vi "Performance Test.vi"() -> ()   [LabVIEW 2021]
uses:
  CIFChannels/Typedef/Direction.ctl
  CIF_NIChn_Fifo_Power.lvclass
  D:/dev/Packages/Channel_Manager/src/CIFChannels/CIFChannels.lvclass
  D:/dev/Packages/Channel_Manager/src/CIF_NIChn/NIChn/CIF_NIChn.lvclass
  ChannelCommon/typedef/FIFO Config.ctl
  <vilib>/Platform/TimedLoop/XDataNode/timing_clust.ctl
  <vilib>/Platform/TimedLoop/XDataNode/nitl_modes.ctl
  <vilib>/Platform/TimedLoop/XDataNode/wakeup.ctl
  ChannelCommon/typedef/Datatype Waveform.ctl
  ChannelCommon/typedef/TimeStamps.ctl
  CIF_NIChn_Fifo_Power.lvclass/CIF_NIChn_Fifo_Power.ctl
  CIFChannels/CIFChannels.lvclass/CIFChannels.ctl
  NIChn/CIF_NIChn.lvclass/CIF_NIChn.ctl
  <vilib>/CIF Foundation/CIF Utilities/DataTypes/Flatten U64.vi
  SubVIs/Add Error.vi
  <vilib>/CIFChannels/Top Level/Write Variable Length U8 Array.vi
  NIChn/Accessors/Read CIF Channel.vi
  NIChn/Accessors/Write CIF Channel.vi
  SubVIs/Flatten.vi
  CIFChannels/Accessors/Read FIFO Payload Length.vi
  NIChn/SubVIs/Check Disconnect.vi
  <vilib>/CIFChannels/Top Level/Read Variable Length U8 Array.vi
  SubVIs/Unflatten.vi
  CIFChannels/Accessors/Read Channel State.vi
  CIFChannels/Accessors/Read Direction.vi
  <vilib>/CIF Foundation/CIF Utilities/Errors/Append Error Location.vi
  <vilib>/CIFChannels/SubVIs/Get dll Path.vi
  ChannelCommon/CIFFIFO/Flatten/Waveform Flatten.vi
  CIFChannels/Accessors/Write Channel State.vi
  CIFChannels/Accessors/Read Tag Disconnect Behavior.vi
  <vilib>/CIFChannels/Top Level/Read Variable Length U8 Array.vi/81056090-23cf-424a-a716-29db01c8ef1b.vi
  <vilib>/CIFChannels/Top Level/Read Variable Length U8 Array.vi/93d598b0-524b-4f76-9570-a74a86ef2c6f.vi
  <vilib>/CIF Foundation/CIF Utilities/DataTypes/Unflatten U64.vi
  ChannelCommon/CIFFIFO/Flatten/Waveform Unflatten.vi
  CIFChannels/Accessors/Write FIFO Header.vi
  CIFChannels/Accessors/Write FIFO Timeout.vi
  <vilib>/CIF Foundation/CIF Utilities/DataTypes/Flatten I64.vi
  ChannelCommon/CIFFIFO/Flatten/Waveform Flatten.vi/be24e584-1bb9-4ddb-b1ad-5fa4498d0a1e.vi
  CIFChannels/Utilities/Create Flattened FIFO Header.vi
  <vilib>/CIFChannels/Top Level/Read Variable Length U8 Array.vi/81056090-23cf-424a-a716-29db01c8ef1b.vi/4bc1c15b-36ab-481f-b8dd-c64075ce723a.vi
  <vilib>/CIFChannels/Top Level/Read Variable Length U8 Array.vi/81056090-23cf-424a-a716-29db01c8ef1b.vi/d83cb72b-7713-41fc-a3d1-682de79cf574.vi
  <vilib>/CIFChannels/Top Level/Read Variable Length U8 Array.vi/93d598b0-524b-4f76-9570-a74a86ef2c6f.vi/4bc1c15b-36ab-481f-b8dd-c64075ce723a.vi
  <vilib>/CIFChannels/Top Level/Read Variable Length U8 Array.vi/93d598b0-524b-4f76-9570-a74a86ef2c6f.vi/d83cb72b-7713-41fc-a3d1-682de79cf574.vi
  ChannelCommon/Utilities/Unflatten Header.vi
  <vilib>/CIF Foundation/CIF Utilities/DataTypes/Unflatten I64.vi
  ChannelCommon/CIFFIFO/Flatten/Waveform Flatten.vi/be24e584-1bb9-4ddb-b1ad-5fa4498d0a1e.vi/c28b0ead-42ad-4072-80a2-aca7f2bd7ce3.vi
  ChannelCommon/Utilities/Flatten Header.vi
  CIFChannels/Utilities/Update FIFO Header.vi
  ChannelCommon/Utilities/Add Error.vi
  <vilib>/CIF Foundation/CIF Utilities/Time/System Time/Get System Time.vi
  <vilib>/CIF Foundation/CIF Utilities/Time/System Time/LabVIEW Time to TAI Time.vi
  NIChn/CIF_NIChn.lvclass
  <vilib>/Platform/TimedLoop/XDataNode/XDataNode.xnode
  <vilib>/Platform/TimedLoop/XDataNode/XDNodeRunTimeDep.lvlib
  CIFChannels/CIFChannels.lvclass
  ChannelCommon/ChannelCommon.lvlib
panel:
  out "avg big channel":dbl
  out "max big channel":dbl
  out "timed out? 4":bool
  out "avg TO":dbl
  out "max TO":dbl
  out "timed out? 3":bool
  out "avg Direct":dbl
  out "max Direct":dbl
  out "timed out? 2":bool
  out "timed out?":bool
  out "avg channel":dbl
  out "max channel":dbl
  out "pass":bool
  out "error out":errorcluster
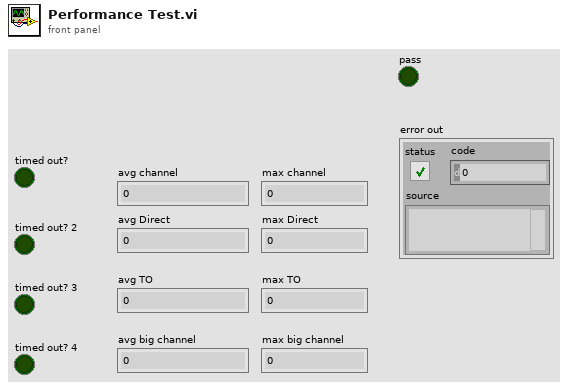
[diagram p1: front panel]
types:
  T1 = typedef "ChannelCommon.lvlib/FIFO Config.ctl" = cluster{"Max Bytes/Msg":u64, "Max Msg/FIFO":u64, "Flags":u64}
  T2 = typedef "CIFChannels.lvclass/Direction.ctl" = enum16{"Publisher", "Subscriber"}
  T3 = typedef "ChannelCommon.lvlib/TimeStamps.ctl" = cluster{"ClockID":u8, "T0":i64, "T_Out":i64}
  T4 = typedef "ChannelCommon.lvlib/Datatype Waveform.ctl" = cluster{"measurement":dbl[], "dT":dbl, "Timestamp":i64, "Read Lock":bool}
  T5 = typedef "XDNodeRunTimeDep.lvlib/timing_clust.ctl" = cluster{"Expected End [f-1]":u64, "Actual End [f-1]":u64, "Finished Late? [f-1]":bool, "Expected End [i-1]":u64, "Actual End [i-1]":u64, "Finished Late? [i-1]":bool, "Expected Start [i]":u64, "Actual Start [i]":u64, "Expected Start [f]":u64, "Actual Start [f]":u64, "Source Name":string, "Structure Name":string, "Period":i64, "Deadline":i64, "Offset":i64, "Start":i64, "Priority":i32, "Timeout":i32, "Mode":T6, "Wakeup Reason":T7, "Error":errorcluster, "Source Type":string, "Secondary Source Type":string, "Global End Time":u64, "Global Start Time":u64, "Frame Duration":u64, "Iteration Duration":u64, "Assigned CPU":i32, "I/O Scan Engine Mode":u32}
  T6 = typedef "XDNodeRunTimeDep.lvlib/nitl_modes.ctl" = enum32{"No Change", "Process missed periods, maintain original phase", "Discard missed periods, maintain original phase", "Process missed periods, ignore original phase", "Discard missed periods, ignore original phase"}
  T7 = typedef "XDNodeRunTimeDep.lvlib/wakeup.ctl" = enum32{"Normal", "Aborted", "Asynchronous wakeup", "Timing source error", "Timed loop error", "Timeout"}
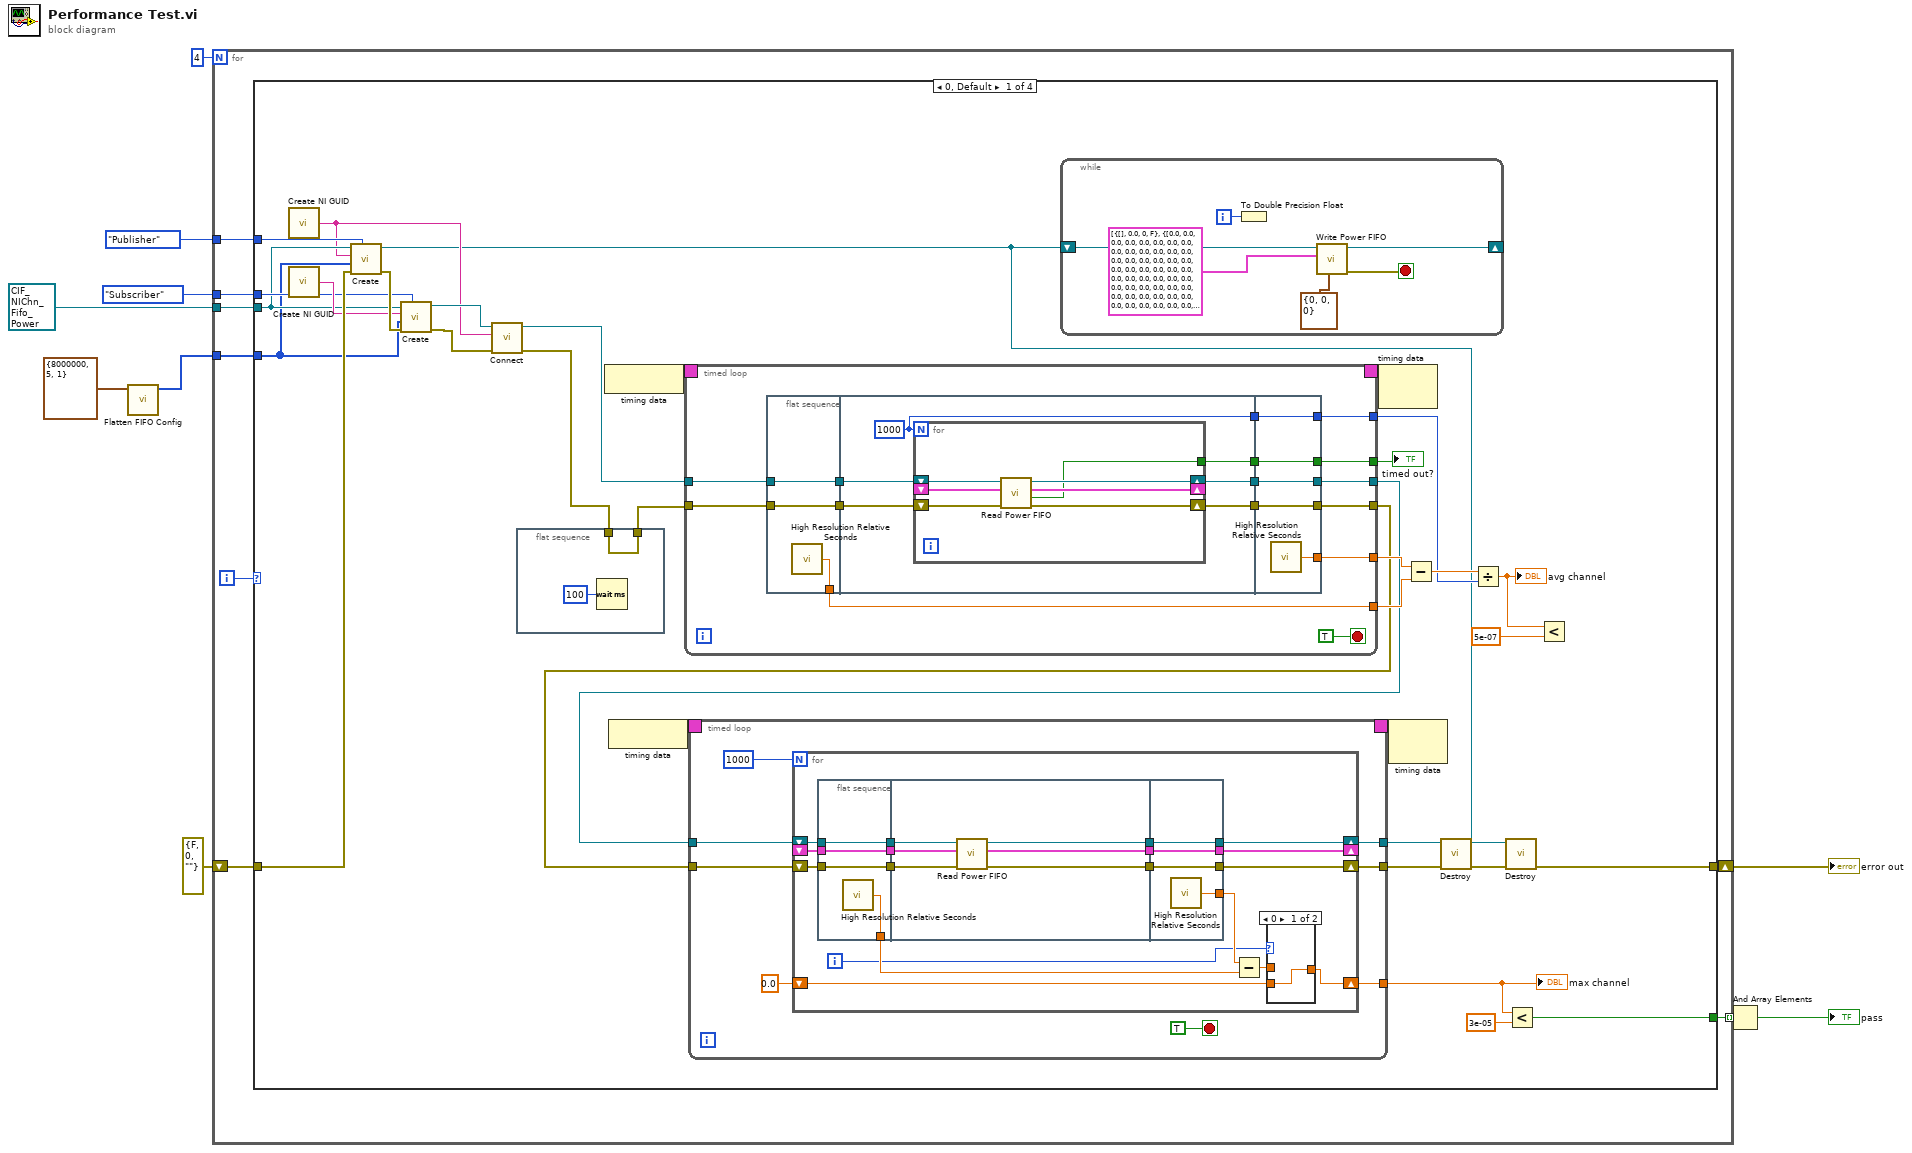
[diagram p0: block diagram]
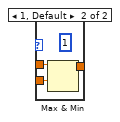
[diagram p2: hidden frame]
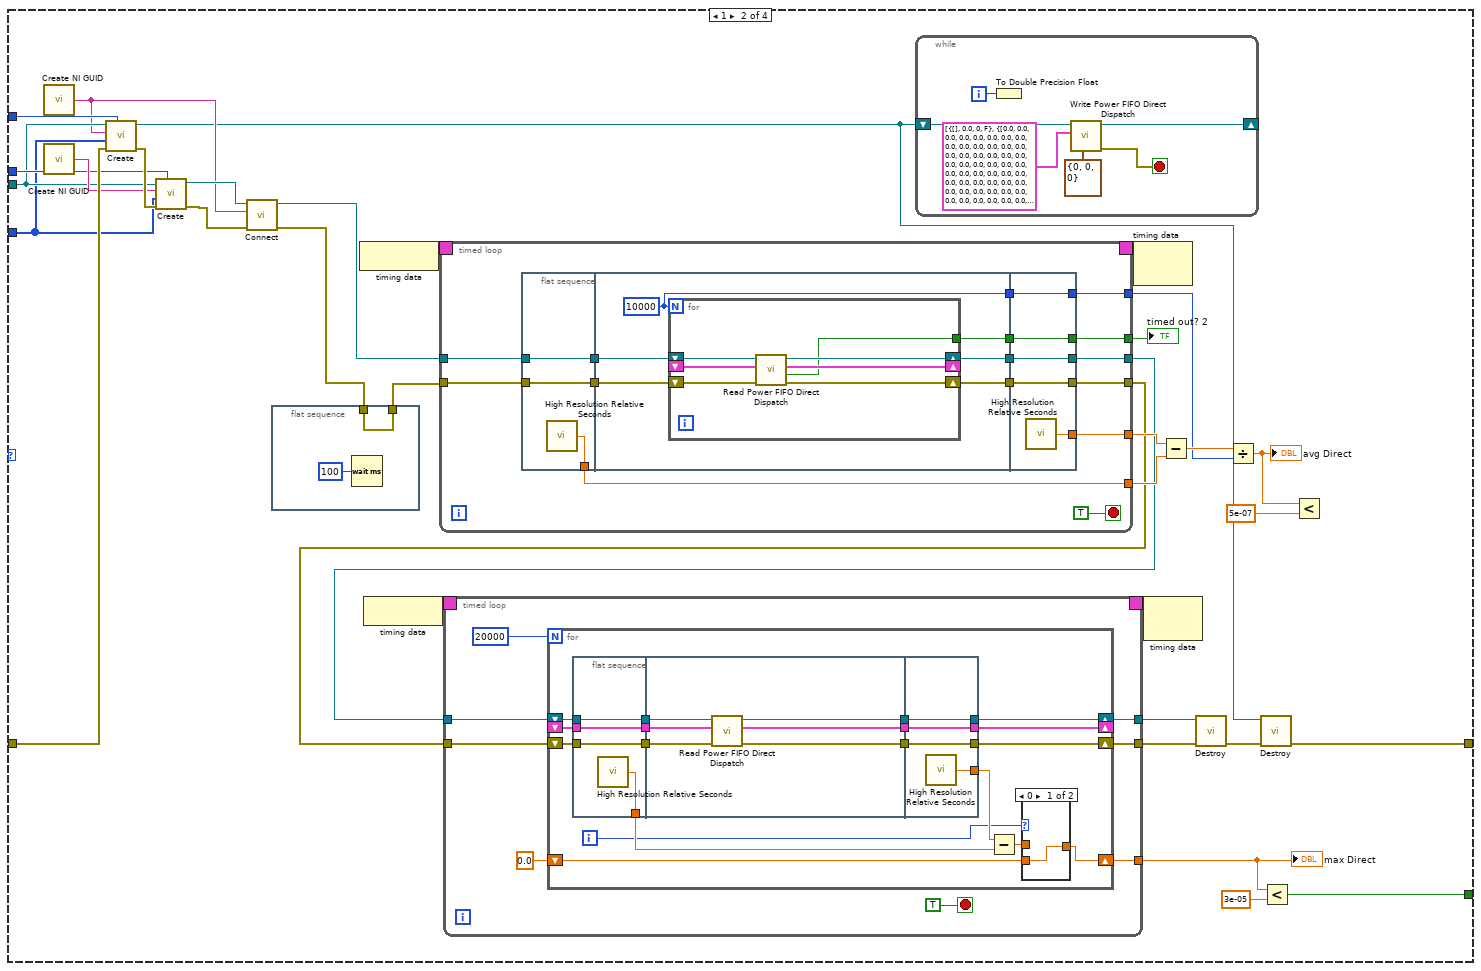
[diagram p3: hidden frame]
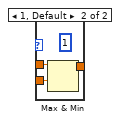
[diagram p4: hidden frame]
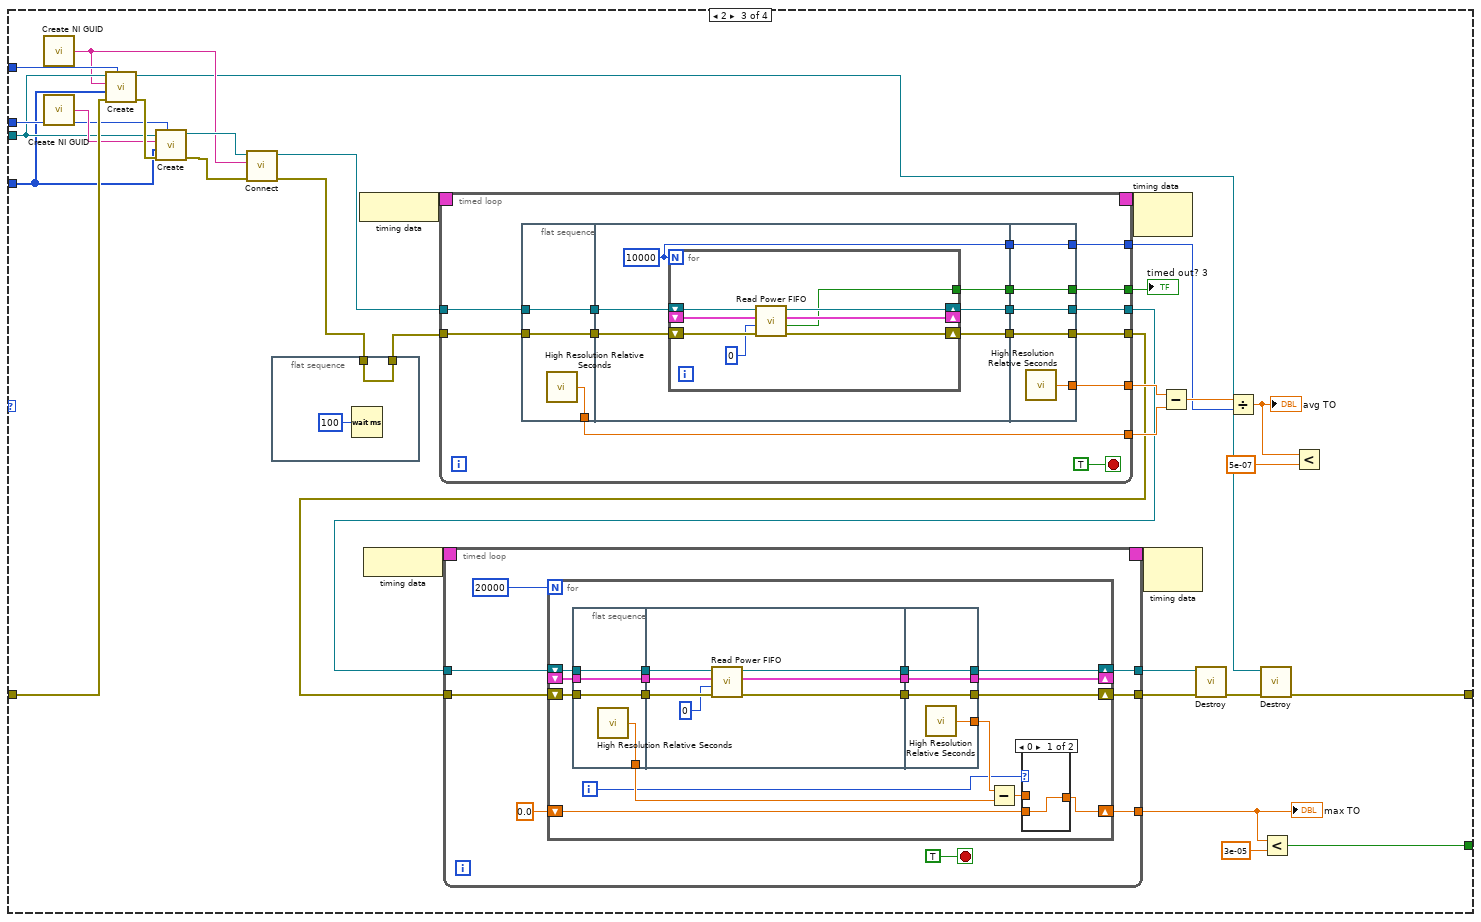
[diagram p5: hidden frame]
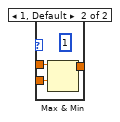
[diagram p6: hidden frame]
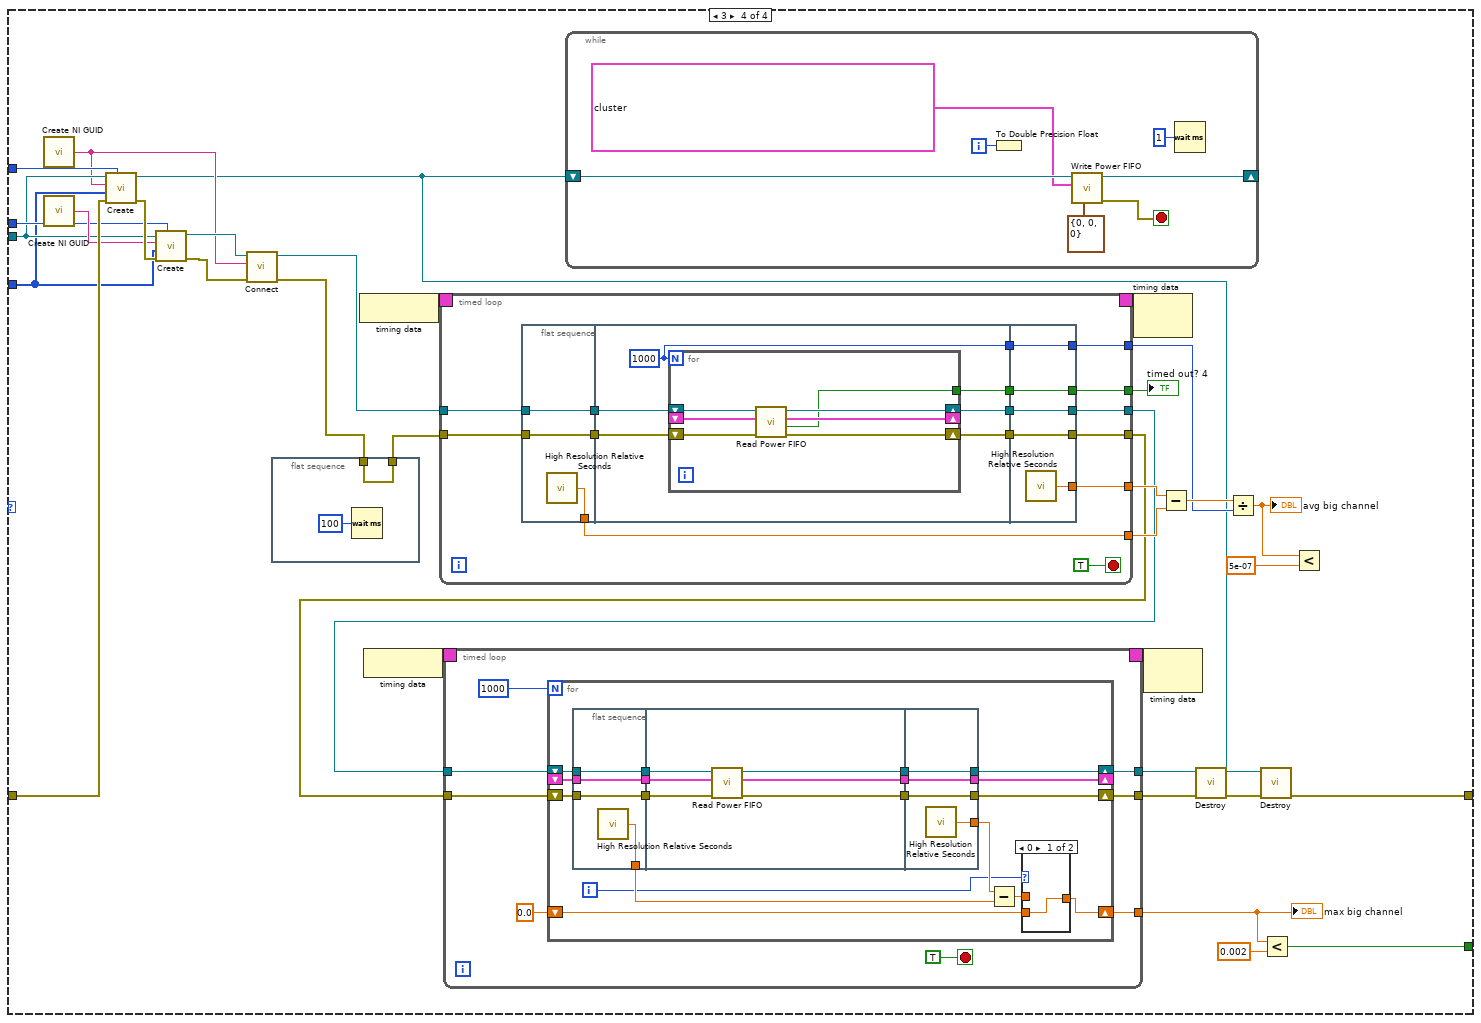
[diagram p7: hidden frame]
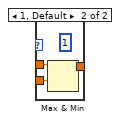
[diagram p8: hidden frame]
diagram:
  n1 = call "Flatten FIFO Config.vi"("FIFO Config in"=T1 {"Max Bytes/Msg"=8000000, "Max Msg/FIFO"=5, "Flags"=1}) -> ("Flattened FIFO Config"=w1:u8[])  [unwired: 10 in]
  n2 = for {
    N: 4 -> [_]
    tunnel: [w18] -> w8 mode=indexing
    shift-right: [w17] -> w10
    shift-left: errorcluster {"status"=FALSE, "code"=0, "source"=""} ("error out") -> [w15]
    tunnel: Direction."Publisher" ("Direction") -> [w14]
    tunnel: Direction."Subscriber" ("Direction") -> [w13]
    tunnel: refnum<class "CIF_NIChn_Fifo_Power.lvclass"> refnum ("CIF_NIChn_Fifo_Power.lvclass") -> [w12]
    tunnel: w1 -> [w11]
    i -> [w16]
    n3 = case shown="0, Default" w16 {
      tunnel: [w38 w168 w298 w424] -> w18
      tunnel: [w22 w152 w282 w408] -> w17
      tunnel: w15 -> [w36 w166 w296 w422]
      tunnel: w14 -> [w34 w164 w294 w420]
      tunnel: w13 -> [w33 w163 w293 w419]
      tunnel: w12 -> [w32 w162 w292 w418]
      tunnel: w11 -> [w28 w158 w288 w414]
      frame 0, Default {
        n4 = call <vilib>:"Create NI GUID.vi"() -> ("NI GUID"=w30:string)
        n5 = call <vilib>:"Create NI GUID.vi"() -> ("NI GUID"=w35:string)
        n6 = call-dynamic "Create.vi"("Direction"=w34, "error in (no error)"=w36, "Custom Config Data"=w28, "Name"=w30, "CIFTag in"=w32) -> ("error out"=w37:errorcluster, "CIFTag out"=w23:refnum<class "CIF_NIChn_Fifo_Power.lvclass">)  [unwired: 5 in]
        n7 = call-dynamic "Create.vi"("Direction"=w33, "error in (no error)"=w37, "Custom Config Data"=w28, "Name"=w35, "CIFTag in"=w32) -> ("error out"=w29:errorcluster, "CIFTag out"=w31:refnum<class "CIF_NIChn_Fifo_Power.lvclass">)  [unwired: 5 in]
        n8 = call-dynamic "Connect.vi"("error in (no error)"=w29, "Connection Name"=w30, "CIFTag in"=w31) -> ("error out"=w21:errorcluster, "CIFTag out"=w27:refnum<class "CIF_NIChn_Fifo_Power.lvclass">)  [unwired: 7 in]
        n9 = flat-sequence {
          tunnel: w21 -> [w54]
          tunnel: [w54] -> w20
          frame #0 {
            n10 = Wait (ms)(milliseconds to wait=u32 100) -> ()  [unwired: 1 out]
          }
        }
        n11 = node-c288() -> (w52:T5)
        n12 = node-c288() -> (w50:T5)
        n13 = timed-loop {
          timing: w52 -> [_]
          timing-out: [_] -> w51
          tunnel: w27 -> [w123]
          tunnel: w20 -> [w122]
          tunnel: [w118] -> w44
          tunnel: [w116] -> w43
          tunnel: [w114] -> w48
          tunnel: [w113] -> w47
          tunnel: [w112] -> w45
          tunnel: [w110] -> w19
          stop <- TRUE stop-if-true
          n14 = flat-sequence {
            tunnel: w122 -> [w125]
            tunnel: w123 -> [w126]
            tunnel: [w126] -> w120
            tunnel: [w125] -> w119
            tunnel: [w124] -> w113
            tunnel: w120 -> [w132]
            tunnel: w119 -> [w131]
            tunnel: [w130] -> w117
            tunnel: [w129] -> w115
            tunnel: [w128] -> w111
            tunnel: [w127] -> w109
            tunnel: [w144] -> w118
            tunnel: w117 -> [w144]
            tunnel: [w143] -> w116
            tunnel: w115 -> [w143]
            tunnel: [w142] -> w114
            tunnel: [w141] -> w112
            tunnel: w111 -> [w141]
            tunnel: [w140] -> w110
            tunnel: w109 -> [w140]
            frame #0 {
              n15 = call <vilib>:"High Resolution Relative Seconds.vi"() -> ("relative seconds"=w124:dbl)
            }
            frame #1 {
              w128 = 1000
              n16 = for {
                N: w128 -> [_]
                shift-right: [w138] -> w130
                shift-left: w132 -> [w139]
                shift-right: [w136] -> w129
                shift-left: w131 -> [w137]
                shift-right: [w135] -> _
                shift-left: _ -> [w133]
                tunnel: [w134] -> w127
                n17 = call-dynamic "Read Power FIFO.vi"("error in (no error)"=w137, "Data in"=w133, "CIFTag in"=w139) -> ("error out"=w136:errorcluster, "timed out?"=w134:bool, "Data out"=w135:T4[], "CIFTag out"=w138:refnum<class "CIF_NIChn_Fifo_Power.lvclass">)  [unwired: 4 in, 1 out]
              }
            }
            frame #2 {
              n18 = call <vilib>:"High Resolution Relative Seconds.vi"() -> ("relative seconds"=w142:dbl)
            }
          }
        }
        "timed out?" <- w19
        n19 = timed-loop {
          timing: w50 -> [_]
          timing-out: [_] -> w49
          tunnel: w44 -> [w68]
          tunnel: w43 -> [w67]
          tunnel: [w65] -> w26
          tunnel: [w64] -> w25
          tunnel: [w61] -> w40
          stop <- TRUE stop-if-true
          n20 = for {
            N: 1000 -> [_]
            shift-right: [w80] -> w65
            shift-left: w68 -> [w82]
            shift-right: [w79] -> w64
            shift-left: w67 -> [w81]
            shift-right: [w73] -> w61
            shift-left: 0.0 -> [w74]
            shift-right: [w72] -> _
            shift-left: _ -> [w78]
            i -> [w70]
            n21 = flat-sequence {
              tunnel: w81 -> [w93]
              tunnel: w82 -> [w94]
              tunnel: [w94] -> w86
              tunnel: [w93] -> w85
              tunnel: [w92] -> w76
              tunnel: w78 -> [w91]
              tunnel: [w91] -> w84
              tunnel: w86 -> [w100]
              tunnel: w85 -> [w98]
              tunnel: [w99] -> w83
              tunnel: w84 -> [w95]
              tunnel: [w96] -> w71
              tunnel: [w97] -> w69
              tunnel: [w104] -> w80
              tunnel: w83 -> [w104]
              tunnel: [w103] -> w79
              tunnel: [w102] -> w77
              tunnel: [w101] -> w72
              tunnel: w71 -> [w101]
              tunnel: w69 -> [w103]
              frame #0 {
                n22 = call <vilib>:"High Resolution Relative Seconds.vi"() -> ("relative seconds"=w92:dbl)
              }
              frame #1 {
                n23 = call-dynamic "Read Power FIFO.vi"("error in (no error)"=w98, "Data in"=w95, "CIFTag in"=w100) -> ("error out"=w97:errorcluster, "Data out"=w96:T4[], "CIFTag out"=w99:refnum<class "CIF_NIChn_Fifo_Power.lvclass">)  [unwired: 4 in, 2 out]
              }
              frame #2 {
                n24 = call <vilib>:"High Resolution Relative Seconds.vi"() -> ("relative seconds"=w102:dbl)
              }
            }
            n25 = Subtract(x=w77, y=w76) -> (x-y=w75:dbl)
            n26 = case shown="0" w70 {
              tunnel: w75 -> [_ w90]
              tunnel: w74 -> [w87 w89]
              tunnel: [w87 w88] -> w73
              frame 0 {
              }
              frame 1, Default {
                (unwired) u32 1 ("milliseconds to wait")
                n27 = Max & Min(x=w90, y=w89) -> (max(x,y)=w88:dbl)  [unwired: 1 out]
              }
            }
          }
        }
        "max channel" <- w40
        n28 = while {
          shift-right: [w55] -> _
          shift-left: w23 -> [w59]
          i -> [w60]
          stop <- w58 stop-if-true
          n29 = To Double Precision Float(number=w60) -> ()  [unwired: 1 out]
          n30 = call-dynamic "Write Power FIFO.vi"("FIFO Timestamps"=T3 {"ClockID"=0, "T0"=0, "T_Out"=0}, "Data In"=T4[] [{"measurement"=[], "dT"=0.0, "Timestamp"=0, "Read Lock"=FALSE}, {"measurement"=[0.0, 0.0, 0.0, 0.0, 0.0, 0.0, 0.0, 0.0, 0.0, 0.0, 0.0, 0.0, 0.0, 0.0, 0.0, 0.0, 0.0, 0.0, 0.0, 0.0, 0.0, 0.0, 0.0, 0.0, 0.0, 0.0, 0.0, 0.0, 0.0, 0.0, 0.0, 0.0, 0.0, 0.0, 0.0, 0.0, 0.0, 0.0, 0.0, 0.0, 0.0, 0.0, 0.0, 0.0, 0.0, 0.0, 0.0, 0.0, 0.0, 0.0, 3.14], "dT"=5.2, "Timestamp"=523, "Read Lock"=FALSE}], "CIFTag in"=w59) -> ("error out"=w58:errorcluster, "CIFTag out"=w55:refnum<class "CIF_NIChn_Fifo_Power.lvclass">)  [unwired: 5 in, 2 out]
        }
        n31 = node-c288(w51) -> ()  [unwired: 1 out]
        n32 = node-c288(w49) -> ()  [unwired: 1 out]
        n33 = Subtract(x=w48, y=w47) -> (x-y=w46:dbl)
        n34 = call-dynamic "Destroy.vi"("error in (no error)"=w25, "CIFTag in"=w26) -> ("error out"=w24:errorcluster)  [unwired: 8 in, 1 out]
        n35 = Divide(x=w46, y=w45) -> (x/y=w42:dbl)
        "avg channel" <- w42
        n36 = call-dynamic "Destroy.vi"("error in (no error)"=w24, "CIFTag in"=w23) -> ("error out"=w22:errorcluster)  [unwired: 8 in, 1 out]
        n37 = Less?(x=w40, y=3e-05) -> (x < y?=w38:bool)
        n38 = Less?(x=w42, y=5e-07) -> ()  [unwired: 1 out]
      }
      frame 1 {
        n39 = call <vilib>:"Create NI GUID.vi"() -> ("NI GUID"=w160:string)
        n40 = call <vilib>:"Create NI GUID.vi"() -> ("NI GUID"=w165:string)
        n41 = call-dynamic "Create.vi"("Direction"=w164, "error in (no error)"=w166, "Custom Config Data"=w158, "Name"=w160, "CIFTag in"=w162) -> ("error out"=w167:errorcluster, "CIFTag out"=w153:refnum<class "CIF_NIChn_Fifo_Power.lvclass">)  [unwired: 5 in]
        n42 = call-dynamic "Create.vi"("Direction"=w163, "error in (no error)"=w167, "Custom Config Data"=w158, "Name"=w165, "CIFTag in"=w162) -> ("error out"=w159:errorcluster, "CIFTag out"=w161:refnum<class "CIF_NIChn_Fifo_Power.lvclass">)  [unwired: 5 in]
        n43 = call-dynamic "Connect.vi"("error in (no error)"=w159, "Connection Name"=w160, "CIFTag in"=w161) -> ("error out"=w151:errorcluster, "CIFTag out"=w157:refnum<class "CIF_NIChn_Fifo_Power.lvclass">)  [unwired: 7 in]
        n44 = flat-sequence {
          tunnel: w151 -> [w184]
          tunnel: [w184] -> w150
          frame #0 {
            n45 = Wait (ms)(milliseconds to wait=u32 100) -> ()  [unwired: 1 out]
          }
        }
        n46 = node-c288() -> (w182:T5)
        n47 = node-c288() -> (w180:T5)
        n48 = timed-loop {
          timing: w182 -> [_]
          timing-out: [_] -> w181
          tunnel: w157 -> [w253]
          tunnel: w150 -> [w252]
          tunnel: [w248] -> w174
          tunnel: [w246] -> w173
          tunnel: [w244] -> w178
          tunnel: [w243] -> w177
          tunnel: [w242] -> w175
          tunnel: [w240] -> w149
          stop <- TRUE stop-if-true
          n49 = flat-sequence {
            tunnel: w252 -> [w255]
            tunnel: w253 -> [w256]
            tunnel: [w256] -> w250
            tunnel: [w255] -> w249
            tunnel: [w254] -> w243
            tunnel: w250 -> [w262]
            tunnel: w249 -> [w261]
            tunnel: [w260] -> w247
            tunnel: [w259] -> w245
            tunnel: [w258] -> w241
            tunnel: [w257] -> w239
            tunnel: [w274] -> w248
            tunnel: w247 -> [w274]
            tunnel: [w273] -> w246
            tunnel: w245 -> [w273]
            tunnel: [w272] -> w244
            tunnel: [w271] -> w242
            tunnel: w241 -> [w271]
            tunnel: [w270] -> w240
            tunnel: w239 -> [w270]
            frame #0 {
              n50 = call <vilib>:"High Resolution Relative Seconds.vi"() -> ("relative seconds"=w254:dbl)
            }
            frame #1 {
              w258 = 10000
              n51 = for {
                N: w258 -> [_]
                shift-right: [w268] -> w260
                shift-left: w262 -> [w269]
                shift-right: [w266] -> w259
                shift-left: w261 -> [w267]
                shift-right: [w265] -> _
                shift-left: _ -> [w263]
                tunnel: [w264] -> w257
                n52 = call "Read Power FIFO Direct Dispatch.vi"("error in (no error)"=w267, "Data in"=w263, "CIFTag in"=w269) -> ("error out"=w266:errorcluster, "timed out?"=w264:bool, "Data out"=w265:T4[], "CIFTag out"=w268:refnum<class "CIF_NIChn_Fifo_Power.lvclass">)  [unwired: 4 in, 1 out]
              }
            }
            frame #2 {
              n53 = call <vilib>:"High Resolution Relative Seconds.vi"() -> ("relative seconds"=w272:dbl)
            }
          }
        }
        "timed out? 2" <- w149
        n54 = timed-loop {
          timing: w180 -> [_]
          timing-out: [_] -> w179
          tunnel: w174 -> [w198]
          tunnel: w173 -> [w197]
          tunnel: [w195] -> w156
          tunnel: [w194] -> w155
          tunnel: [w191] -> w170
          stop <- TRUE stop-if-true
          n55 = for {
            N: 20000 -> [_]
            shift-right: [w210] -> w195
            shift-left: w198 -> [w212]
            shift-right: [w209] -> w194
            shift-left: w197 -> [w211]
            shift-right: [w203] -> w191
            shift-left: 0.0 -> [w204]
            shift-right: [w202] -> _
            shift-left: _ -> [w208]
            i -> [w200]
            n56 = flat-sequence {
              tunnel: w211 -> [w223]
              tunnel: w212 -> [w224]
              tunnel: [w224] -> w216
              tunnel: [w223] -> w215
              tunnel: [w222] -> w206
              tunnel: w208 -> [w221]
              tunnel: [w221] -> w214
              tunnel: w216 -> [w230]
              tunnel: w215 -> [w228]
              tunnel: [w229] -> w213
              tunnel: w214 -> [w225]
              tunnel: [w226] -> w201
              tunnel: [w227] -> w199
              tunnel: [w234] -> w210
              tunnel: w213 -> [w234]
              tunnel: [w233] -> w209
              tunnel: [w232] -> w207
              tunnel: [w231] -> w202
              tunnel: w201 -> [w231]
              tunnel: w199 -> [w233]
              frame #0 {
                n57 = call <vilib>:"High Resolution Relative Seconds.vi"() -> ("relative seconds"=w222:dbl)
              }
              frame #1 {
                n58 = call "Read Power FIFO Direct Dispatch.vi"("error in (no error)"=w228, "Data in"=w225, "CIFTag in"=w230) -> ("error out"=w227:errorcluster, "Data out"=w226:T4[], "CIFTag out"=w229:refnum<class "CIF_NIChn_Fifo_Power.lvclass">)  [unwired: 4 in, 2 out]
              }
              frame #2 {
                n59 = call <vilib>:"High Resolution Relative Seconds.vi"() -> ("relative seconds"=w232:dbl)
              }
            }
            n60 = Subtract(x=w207, y=w206) -> (x-y=w205:dbl)
            n61 = case shown="0" w200 {
              tunnel: w205 -> [_ w220]
              tunnel: w204 -> [w217 w219]
              tunnel: [w217 w218] -> w203
              frame 0 {
              }
              frame 1, Default {
                (unwired) u32 1 ("milliseconds to wait")
                n62 = Max & Min(x=w220, y=w219) -> (max(x,y)=w218:dbl)  [unwired: 1 out]
              }
            }
          }
        }
        "max Direct" <- w170
        n63 = while {
          shift-right: [w185] -> _
          shift-left: w153 -> [w189]
          i -> [w190]
          stop <- w188 stop-if-true
          n64 = To Double Precision Float(number=w190) -> ()  [unwired: 1 out]
          n65 = call "Write Power FIFO Direct Dispatch.vi"("FIFO Timestamps"=T3 {"ClockID"=0, "T0"=0, "T_Out"=0}, "Data In"=T4[] [{"measurement"=[], "dT"=0.0, "Timestamp"=0, "Read Lock"=FALSE}, {"measurement"=[0.0, 0.0, 0.0, 0.0, 0.0, 0.0, 0.0, 0.0, 0.0, 0.0, 0.0, 0.0, 0.0, 0.0, 0.0, 0.0, 0.0, 0.0, 0.0, 0.0, 0.0, 0.0, 0.0, 0.0, 0.0, 0.0, 0.0, 0.0, 0.0, 0.0, 0.0, 0.0, 0.0, 0.0, 0.0, 0.0, 0.0, 0.0, 0.0, 0.0, 0.0, 0.0, 0.0, 0.0, 0.0, 0.0, 0.0, 0.0, 0.0, 0.0, 3.14], "dT"=5.2, "Timestamp"=523, "Read Lock"=FALSE}], "CIFTag in"=w189) -> ("error out"=w188:errorcluster, "CIFTag out"=w185:refnum<class "CIF_NIChn_Fifo_Power.lvclass">)  [unwired: 5 in, 2 out]
        }
        n66 = node-c288(w181) -> ()  [unwired: 1 out]
        n67 = node-c288(w179) -> ()  [unwired: 1 out]
        n68 = Subtract(x=w178, y=w177) -> (x-y=w176:dbl)
        n69 = call-dynamic "Destroy.vi"("error in (no error)"=w155, "CIFTag in"=w156) -> ("error out"=w154:errorcluster)  [unwired: 8 in, 1 out]
        n70 = Divide(x=w176, y=w175) -> (x/y=w172:dbl)
        "avg Direct" <- w172
        n71 = call-dynamic "Destroy.vi"("error in (no error)"=w154, "CIFTag in"=w153) -> ("error out"=w152:errorcluster)  [unwired: 8 in, 1 out]
        n72 = Less?(x=w170, y=3e-05) -> (x < y?=w168:bool)
        n73 = Less?(x=w172, y=5e-07) -> ()  [unwired: 1 out]
      }
      frame 2 {
        n74 = call <vilib>:"Create NI GUID.vi"() -> ("NI GUID"=w290:string)
        n75 = call <vilib>:"Create NI GUID.vi"() -> ("NI GUID"=w295:string)
        n76 = call-dynamic "Create.vi"("Direction"=w294, "error in (no error)"=w296, "Custom Config Data"=w288, "Name"=w290, "CIFTag in"=w292) -> ("error out"=w297:errorcluster, "CIFTag out"=w283:refnum<class "CIF_NIChn_Fifo_Power.lvclass">)  [unwired: 5 in]
        n77 = call-dynamic "Create.vi"("Direction"=w293, "error in (no error)"=w297, "Custom Config Data"=w288, "Name"=w295, "CIFTag in"=w292) -> ("error out"=w289:errorcluster, "CIFTag out"=w291:refnum<class "CIF_NIChn_Fifo_Power.lvclass">)  [unwired: 5 in]
        n78 = call-dynamic "Connect.vi"("error in (no error)"=w289, "Connection Name"=w290, "CIFTag in"=w291) -> ("error out"=w281:errorcluster, "CIFTag out"=w287:refnum<class "CIF_NIChn_Fifo_Power.lvclass">)  [unwired: 7 in]
        n79 = flat-sequence {
          tunnel: w281 -> [w314]
          tunnel: [w314] -> w280
          frame #0 {
            n80 = Wait (ms)(milliseconds to wait=u32 100) -> ()  [unwired: 1 out]
          }
        }
        n81 = node-c288() -> (w312:T5)
        n82 = node-c288() -> (w310:T5)
        n83 = timed-loop {
          timing: w312 -> [_]
          timing-out: [_] -> w311
          tunnel: w287 -> [w378]
          tunnel: w280 -> [w377]
          tunnel: [w373] -> w304
          tunnel: [w371] -> w303
          tunnel: [w369] -> w308
          tunnel: [w368] -> w307
          tunnel: [w367] -> w305
          tunnel: [w365] -> w279
          stop <- TRUE stop-if-true
          n84 = flat-sequence {
            tunnel: w377 -> [w380]
            tunnel: w378 -> [w381]
            tunnel: [w381] -> w375
            tunnel: [w380] -> w374
            tunnel: [w379] -> w368
            tunnel: w375 -> [w387]
            tunnel: w374 -> [w386]
            tunnel: [w385] -> w372
            tunnel: [w384] -> w370
            tunnel: [w383] -> w366
            tunnel: [w382] -> w364
            tunnel: [w400] -> w373
            tunnel: w372 -> [w400]
            tunnel: [w399] -> w371
            tunnel: w370 -> [w399]
            tunnel: [w398] -> w369
            tunnel: [w397] -> w367
            tunnel: w366 -> [w397]
            tunnel: [w396] -> w365
            tunnel: w364 -> [w396]
            frame #0 {
              n85 = call <vilib>:"High Resolution Relative Seconds.vi"() -> ("relative seconds"=w379:dbl)
            }
            frame #1 {
              w383 = 10000
              n86 = for {
                N: w383 -> [_]
                shift-right: [w394] -> w385
                shift-left: w387 -> [w395]
                shift-right: [w392] -> w384
                shift-left: w386 -> [w393]
                shift-right: [w391] -> _
                shift-left: _ -> [w388]
                tunnel: [w390] -> w382
                n87 = call-dynamic "Read Power FIFO.vi"("error in (no error)"=w393, "Timeout (ms)"=0, "Data in"=w388, "CIFTag in"=w395) -> ("error out"=w392:errorcluster, "timed out?"=w390:bool, "Data out"=w391:T4[], "CIFTag out"=w394:refnum<class "CIF_NIChn_Fifo_Power.lvclass">)  [unwired: 3 in, 1 out]
              }
            }
            frame #2 {
              n88 = call <vilib>:"High Resolution Relative Seconds.vi"() -> ("relative seconds"=w398:dbl)
            }
          }
        }
        "timed out? 3" <- w279
        n89 = timed-loop {
          timing: w310 -> [_]
          timing-out: [_] -> w309
          tunnel: w304 -> [w322]
          tunnel: w303 -> [w321]
          tunnel: [w319] -> w286
          tunnel: [w318] -> w285
          tunnel: [w315] -> w300
          stop <- TRUE stop-if-true
          n90 = for {
            N: 20000 -> [_]
            shift-right: [w334] -> w319
            shift-left: w322 -> [w336]
            shift-right: [w333] -> w318
            shift-left: w321 -> [w335]
            shift-right: [w327] -> w315
            shift-left: 0.0 -> [w328]
            shift-right: [w326] -> _
            shift-left: _ -> [w332]
            i -> [w324]
            n91 = flat-sequence {
              tunnel: w335 -> [w347]
              tunnel: w336 -> [w348]
              tunnel: [w348] -> w340
              tunnel: [w347] -> w339
              tunnel: [w346] -> w330
              tunnel: w332 -> [w345]
              tunnel: [w345] -> w338
              tunnel: w340 -> [w355]
              tunnel: w339 -> [w353]
              tunnel: [w354] -> w337
              tunnel: w338 -> [w349]
              tunnel: [w351] -> w325
              tunnel: [w352] -> w323
              tunnel: [w359] -> w334
              tunnel: w337 -> [w359]
              tunnel: [w358] -> w333
              tunnel: [w357] -> w331
              tunnel: [w356] -> w326
              tunnel: w325 -> [w356]
              tunnel: w323 -> [w358]
              frame #0 {
                n92 = call <vilib>:"High Resolution Relative Seconds.vi"() -> ("relative seconds"=w346:dbl)
              }
              frame #1 {
                n93 = call-dynamic "Read Power FIFO.vi"("error in (no error)"=w353, "Timeout (ms)"=0, "Data in"=w349, "CIFTag in"=w355) -> ("error out"=w352:errorcluster, "Data out"=w351:T4[], "CIFTag out"=w354:refnum<class "CIF_NIChn_Fifo_Power.lvclass">)  [unwired: 3 in, 2 out]
              }
              frame #2 {
                n94 = call <vilib>:"High Resolution Relative Seconds.vi"() -> ("relative seconds"=w357:dbl)
              }
            }
            n95 = Subtract(x=w331, y=w330) -> (x-y=w329:dbl)
            n96 = case shown="0" w324 {
              tunnel: w329 -> [_ w344]
              tunnel: w328 -> [w341 w343]
              tunnel: [w341 w342] -> w327
              frame 0 {
              }
              frame 1, Default {
                (unwired) u32 1 ("milliseconds to wait")
                n97 = Max & Min(x=w344, y=w343) -> (max(x,y)=w342:dbl)  [unwired: 1 out]
              }
            }
          }
        }
        "max TO" <- w300
        n98 = node-c288(w311) -> ()  [unwired: 1 out]
        n99 = node-c288(w309) -> ()  [unwired: 1 out]
        n100 = Subtract(x=w308, y=w307) -> (x-y=w306:dbl)
        n101 = call-dynamic "Destroy.vi"("error in (no error)"=w285, "CIFTag in"=w286) -> ("error out"=w284:errorcluster)  [unwired: 8 in, 1 out]
        n102 = Divide(x=w306, y=w305) -> (x/y=w302:dbl)
        "avg TO" <- w302
        n103 = call-dynamic "Destroy.vi"("error in (no error)"=w284, "CIFTag in"=w283) -> ("error out"=w282:errorcluster)  [unwired: 8 in, 1 out]
        n104 = Less?(x=w300, y=3e-05) -> (x < y?=w298:bool)
        n105 = Less?(x=w302, y=5e-07) -> ()  [unwired: 1 out]
      }
      frame 3 {
        n106 = call <vilib>:"Create NI GUID.vi"() -> ("NI GUID"=w416:string)
        n107 = call <vilib>:"Create NI GUID.vi"() -> ("NI GUID"=w421:string)
        n108 = call-dynamic "Create.vi"("Direction"=w420, "error in (no error)"=w422, "Custom Config Data"=w414, "Name"=w416, "CIFTag in"=w418) -> ("error out"=w423:errorcluster, "CIFTag out"=w409:refnum<class "CIF_NIChn_Fifo_Power.lvclass">)  [unwired: 5 in]
        n109 = call-dynamic "Create.vi"("Direction"=w419, "error in (no error)"=w423, "Custom Config Data"=w414, "Name"=w421, "CIFTag in"=w418) -> ("error out"=w415:errorcluster, "CIFTag out"=w417:refnum<class "CIF_NIChn_Fifo_Power.lvclass">)  [unwired: 5 in]
        n110 = call-dynamic "Connect.vi"("error in (no error)"=w415, "Connection Name"=w416, "CIFTag in"=w417) -> ("error out"=w407:errorcluster, "CIFTag out"=w413:refnum<class "CIF_NIChn_Fifo_Power.lvclass">)  [unwired: 7 in]
        n111 = flat-sequence {
          tunnel: w407 -> [w440]
          tunnel: [w440] -> w406
          frame #0 {
            n112 = Wait (ms)(milliseconds to wait=u32 100) -> ()  [unwired: 1 out]
          }
        }
        n113 = node-c288() -> (w438:T5)
        n114 = node-c288() -> (w436:T5)
        n115 = timed-loop {
          timing: w438 -> [_]
          timing-out: [_] -> w437
          tunnel: w413 -> [w510]
          tunnel: w406 -> [w509]
          tunnel: [w505] -> w430
          tunnel: [w503] -> w429
          tunnel: [w501] -> w434
          tunnel: [w500] -> w433
          tunnel: [w499] -> w431
          tunnel: [w497] -> w405
          stop <- TRUE stop-if-true
          n116 = flat-sequence {
            tunnel: w509 -> [w512]
            tunnel: w510 -> [w513]
            tunnel: [w513] -> w507
            tunnel: [w512] -> w506
            tunnel: [w511] -> w500
            tunnel: w507 -> [w519]
            tunnel: w506 -> [w518]
            tunnel: [w517] -> w504
            tunnel: [w516] -> w502
            tunnel: [w515] -> w498
            tunnel: [w514] -> w496
            tunnel: [w531] -> w505
            tunnel: w504 -> [w531]
            tunnel: [w530] -> w503
            tunnel: w502 -> [w530]
            tunnel: [w529] -> w501
            tunnel: [w528] -> w499
            tunnel: w498 -> [w528]
            tunnel: [w527] -> w497
            tunnel: w496 -> [w527]
            frame #0 {
              n117 = call <vilib>:"High Resolution Relative Seconds.vi"() -> ("relative seconds"=w511:dbl)
            }
            frame #1 {
              w515 = 1000
              n118 = for {
                N: w515 -> [_]
                shift-right: [w525] -> w517
                shift-left: w519 -> [w526]
                shift-right: [w523] -> w516
                shift-left: w518 -> [w524]
                shift-right: [w522] -> _
                shift-left: _ -> [w520]
                tunnel: [w521] -> w514
                n119 = call-dynamic "Read Power FIFO.vi"("error in (no error)"=w524, "Data in"=w520, "CIFTag in"=w526) -> ("error out"=w523:errorcluster, "timed out?"=w521:bool, "Data out"=w522:T4[], "CIFTag out"=w525:refnum<class "CIF_NIChn_Fifo_Power.lvclass">)  [unwired: 4 in, 1 out]
              }
            }
            frame #2 {
              n120 = call <vilib>:"High Resolution Relative Seconds.vi"() -> ("relative seconds"=w529:dbl)
            }
          }
        }
        "timed out? 4" <- w405
        n121 = timed-loop {
          timing: w436 -> [_]
          timing-out: [_] -> w435
          tunnel: w430 -> [w455]
          tunnel: w429 -> [w454]
          tunnel: [w452] -> w412
          tunnel: [w451] -> w411
          tunnel: [w448] -> w426
          stop <- TRUE stop-if-true
          n122 = for {
            N: 1000 -> [_]
            shift-right: [w467] -> w452
            shift-left: w455 -> [w469]
            shift-right: [w466] -> w451
            shift-left: w454 -> [w468]
            shift-right: [w460] -> w448
            shift-left: 0.0 -> [w461]
            shift-right: [w459] -> _
            shift-left: _ -> [w465]
            i -> [w457]
            n123 = flat-sequence {
              tunnel: w468 -> [w480]
              tunnel: w469 -> [w481]
              tunnel: [w481] -> w473
              tunnel: [w480] -> w472
              tunnel: [w479] -> w463
              tunnel: w465 -> [w478]
              tunnel: [w478] -> w471
              tunnel: w473 -> [w487]
              tunnel: w472 -> [w485]
              tunnel: [w486] -> w470
              tunnel: w471 -> [w482]
              tunnel: [w483] -> w458
              tunnel: [w484] -> w456
              tunnel: [w491] -> w467
              tunnel: w470 -> [w491]
              tunnel: [w490] -> w466
              tunnel: [w489] -> w464
              tunnel: [w488] -> w459
              tunnel: w458 -> [w488]
              tunnel: w456 -> [w490]
              frame #0 {
                n124 = call <vilib>:"High Resolution Relative Seconds.vi"() -> ("relative seconds"=w479:dbl)
              }
              frame #1 {
                n125 = call-dynamic "Read Power FIFO.vi"("error in (no error)"=w485, "Data in"=w482, "CIFTag in"=w487) -> ("error out"=w484:errorcluster, "Data out"=w483:T4[], "CIFTag out"=w486:refnum<class "CIF_NIChn_Fifo_Power.lvclass">)  [unwired: 4 in, 2 out]
              }
              frame #2 {
                n126 = call <vilib>:"High Resolution Relative Seconds.vi"() -> ("relative seconds"=w489:dbl)
              }
            }
            n127 = Subtract(x=w464, y=w463) -> (x-y=w462:dbl)
            n128 = case shown="0" w457 {
              tunnel: w462 -> [_ w477]
              tunnel: w461 -> [w474 w476]
              tunnel: [w474 w475] -> w460
              frame 0 {
              }
              frame 1, Default {
                (unwired) u32 1 ("milliseconds to wait")
                n129 = Max & Min(x=w477, y=w476) -> (max(x,y)=w475:dbl)  [unwired: 1 out]
              }
            }
          }
        }
        "max big channel" <- w426
        n130 = while {
          shift-right: [w441] -> _
          shift-left: w409 -> [w446]
          i -> [w447]
          stop <- w445 stop-if-true
          n131 = To Double Precision Float(number=w447) -> ()  [unwired: 1 out]
          n132 = call-dynamic "Write Power FIFO.vi"("FIFO Timestamps"=T3 {"ClockID"=0, "T0"=0, "T_Out"=0}, "Data In"=T4[] [{"measurement"=array[200001 elements], "dT"=0.0, "Timestamp"=0, "Read Lock"=FALSE}, {"measurement"=array[200001 elements], "dT"=5.2, "Timestamp"=523, "Read Lock"=FALSE}], "CIFTag in"=w446) -> ("error out"=w445:errorcluster, "CIFTag out"=w441:refnum<class "CIF_NIChn_Fifo_Power.lvclass">)  [unwired: 5 in, 2 out]
          n133 = Wait (ms)(milliseconds to wait=u32 1) -> ()  [unwired: 1 out]
        }
        n134 = node-c288(w437) -> ()  [unwired: 1 out]
        n135 = node-c288(w435) -> ()  [unwired: 1 out]
        n136 = Subtract(x=w434, y=w433) -> (x-y=w432:dbl)
        n137 = call-dynamic "Destroy.vi"("error in (no error)"=w411, "CIFTag in"=w412) -> ("error out"=w410:errorcluster)  [unwired: 8 in, 1 out]
        n138 = Divide(x=w432, y=w431) -> (x/y=w428:dbl)
        "avg big channel" <- w428
        n139 = call-dynamic "Destroy.vi"("error in (no error)"=w410, "CIFTag in"=w409) -> ("error out"=w408:errorcluster)  [unwired: 8 in, 1 out]
        n140 = Less?(x=w426, y=0.002) -> (x < y?=w424:bool)
        n141 = Less?(x=w428, y=5e-07) -> ()  [unwired: 1 out]
      }
    }
  }
  "error out" <- w10
  n142 = And Array Elements(Boolean array=w8) -> (logical AND=→"pass":bool)
